vi "Current Grabber State.vi"(8 "error in (no error)":errorcluster, 10 "Grabber State":T1, 11 "Grabber in":refnum<class "Grabber.lvclass">) -> (0 "error out":errorcluster, 3 "Grabber out":refnum<class "Grabber.lvclass">)   [LabVIEW 2014, in "Grabber.lvlib" / "Grabber.lvclass"]
uses:
  Grabber.lvclass
  Grabber State.ctl
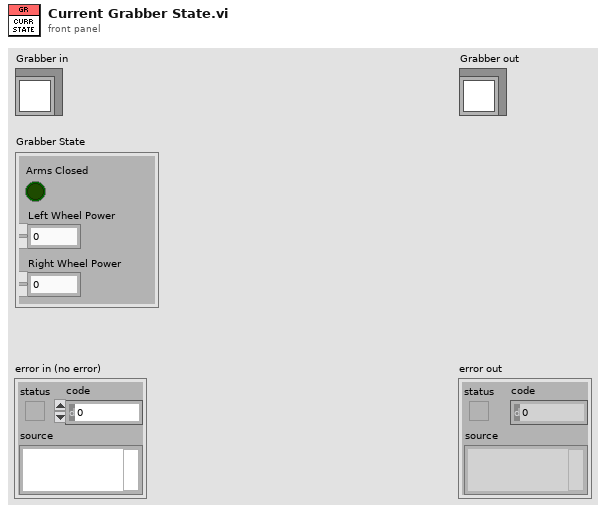
[diagram p1: front panel]
types:
  T1 = typedef "Grabber.lvlib/Grabber.lvclass/Grabber State.ctl" = cluster{"Arms Closed":bool, "Left Wheel Power":dbl, "Right Wheel Power":dbl}
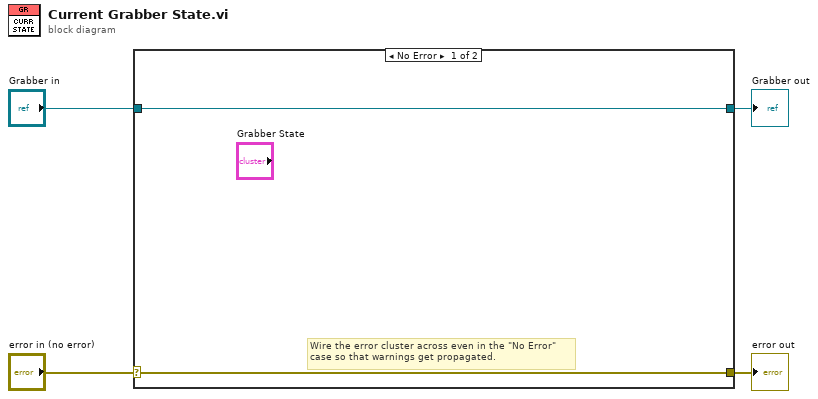
[diagram p0: block diagram]
diagram:
  n1 = case shown="No Error" "error in (no error)" {
    selector: "error in (no error)" -> [w5 w8]
    tunnel: [w5 w8] -> w3
    tunnel: [w6 w7] -> w1
    tunnel: "Grabber in" -> [w6 w7]
    frame No Error {
      # "Wire the error cluster across even in the \"No Error\"\ncase so that warnings get propagated."
    }
    frame Error {
    }
  }
  "error out" <- w3
  "Grabber out" <- w1
